vi "LeapYearSubVI.vi"(1 "Year":i16 min=0 step=1, 2 "Month":i8=1 min=1 max=12 step=1) -> (0 "Leap Year?":bool)   [LabVIEW 2020]
doc: "Requires a numeric (1-12) month and year; returns True if it's a leap year, False if not."
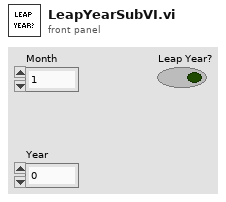
[diagram p1: front panel]
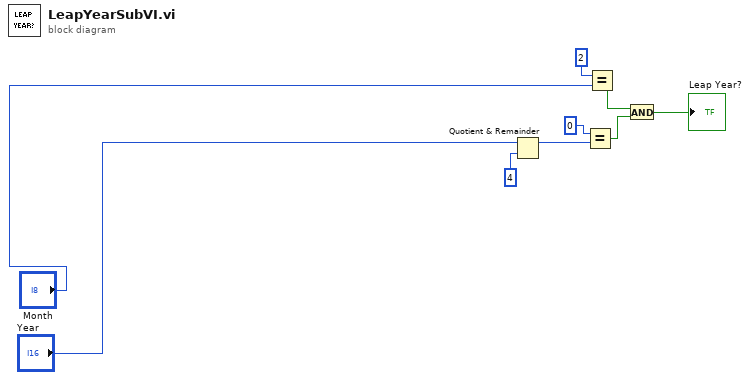
[diagram p0: block diagram]
diagram:
  n1 = Quotient & Remainder(x="Year", y=4) -> (x-y*floor(x/y)=w9:i32)  [unwired: 1 out]
  n2 = Equal?(x=0, y=w9) -> (x = y?=w5:bool)
  n3 = Equal?(x=2, y="Month") -> (x = y?=w1:bool)
  n4 = And(x=w1, y=w5) -> (x .and. y?=→"Leap Year?":bool)
